vi "fgv_loop_count.vi"(7 "cmd":enum16{"init", "read", "write"}(ring), 8 "error in":errorcluster, 11 "loop count in":T1) -> (0 "error out":errorcluster, 3 "loop count out":T1)   [LabVIEW 2019]
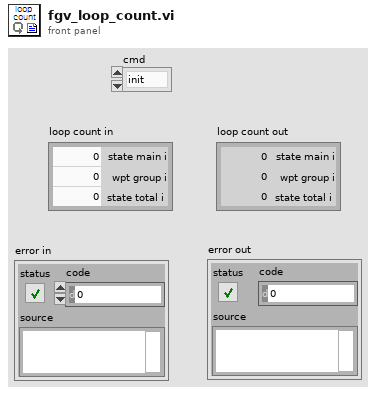
[diagram p1: front panel]
types:
  T1 = cluster{"wpt group i":i32, "state total i":i32, "state main i":i32}
  T2 = cluster{"state total i":i32, "wpt group i":i32, "state main i":i32}
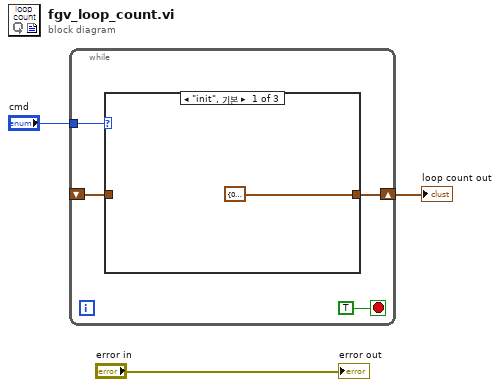
[diagram p0: block diagram]
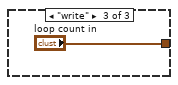
[diagram p3: hidden frame]
diagram:
  n1 = while {
    tunnel: "cmd" -> [w6]
    shift-right: [w5] -> w1
    shift-left: _ -> [w4]
    stop <- TRUE stop-if-true
    n2 = case shown="\"init\", 기본" w6 {
      tunnel: [T2 {"state total i"=0, "wpt group i"=0, "state main i"=0} ("loop data in") w9 "loop count in"] -> w5
      tunnel: w4 -> [_ w9 _]
      frame "init", Default {
      }
      frame "read" {
      }
      frame "write" {
      }
    }
  }
  "loop count out" <- w1
  "error out" <- "error in"
